vi "Click and Drag on .NET Container.vi"() -> ()   [LabVIEW 2014]
uses:
  <vilib>/Utility/miscctls.llb/LVPoint32TypeDef.ctl
panel:
  out "Button":u16
  out "Coords":T1
  in  "Stop Button":bool
  in  ".NET Container":refnum<k24>(container)
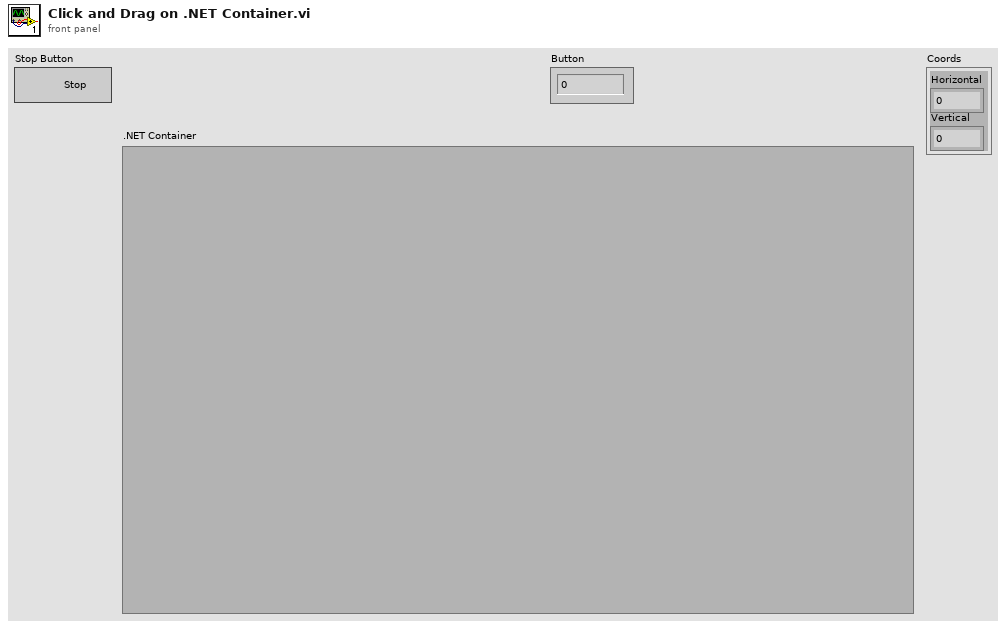
[diagram p1: front panel]
types:
  T1 = typedef "LVPoint32TypeDef.ctl" = cluster{"Horizontal":i32, "Vertical":i32}
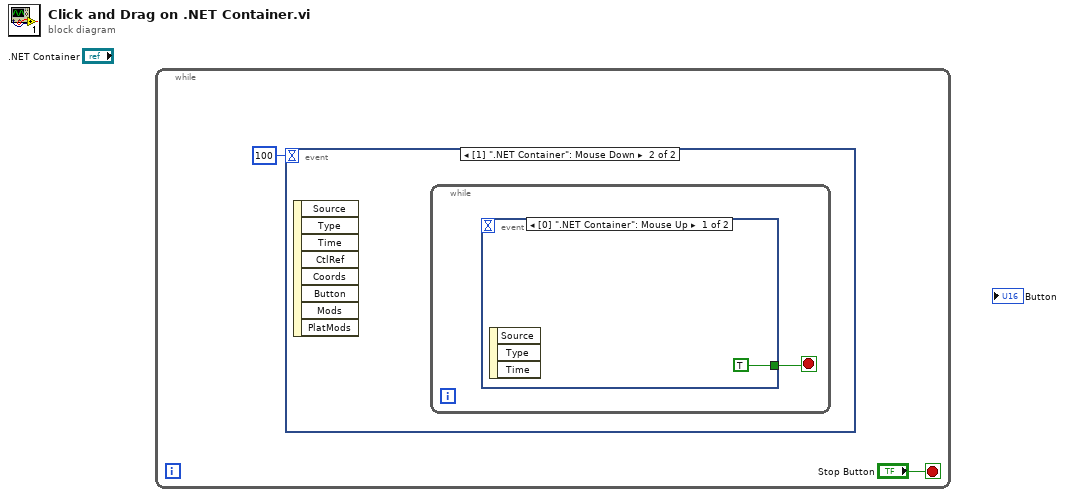
[diagram p0: block diagram]
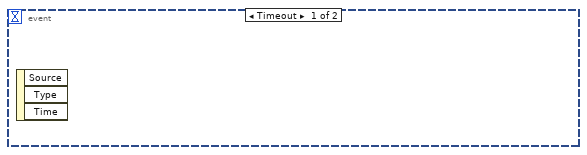
[diagram p2: hidden frame]
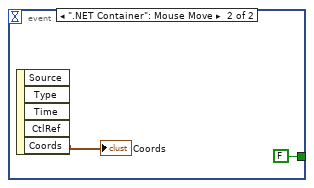
[diagram p3: hidden frame]
diagram:
  n1 = while {
    stop <- "Stop Button" stop-if-true
    n2 = event shown="[1] \".NET Container\": Mouse Down" {
      selector: _ -> [_ _]
      dyn-events: _ -> [_ _]
      timeout: 100 -> [_ _]
      event Timeout {
        n3 = event-data() -> ()  [unwired: 1 in, 3 out]
      }
      event ".NET Container": Mouse Down {
        n4 = event-data() -> ()  [unwired: 1 in, 8 out]
        n5 = while {
          stop <- w3 stop-if-true
          n6 = event shown="[0] \".NET Container\": Mouse Up" {
            selector: _ -> [_ _]
            dyn-events: _ -> [_ _]
            timeout: _ -> [_ _]
            tunnel: [TRUE FALSE] -> w3
            event ".NET Container": Mouse Up {
              n7 = event-data() -> ()  [unwired: 1 in, 3 out]
            }
            event ".NET Container": Mouse Move {
              n8 = event-data() -> ("Coords"=→"Coords":T1)  [unwired: 1 in, 4 out]
            }
          }
        }
      }
    }
  }
